vi "MenuBar Visable.vi"(8 "error in (no error)":errorcluster, 10 "Disabled":T1(ring)=enum."Disabled and Grayed Out", 11 "Main in":refnum<class "Main.lvclass">) -> (0 "error out":errorcluster, 3 "Main out":refnum<class "Main.lvclass">)   [LabVIEW 2023, in "GUI.lvlib" / "Main.lvlib" / "Main.lvclass"]
uses:
  Main.lvclass
  Main.lvclass/Main.ctl
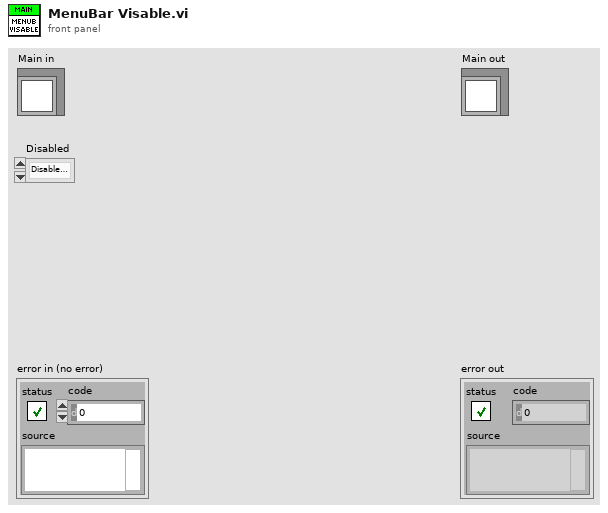
[diagram p1: front panel]
types:
  T1 = enum8{"Enabled", "Disabled", "Disabled and Grayed Out"}
  T2 = typedef "GUI.lvlib/Main.App.Cluster.ctl" = cluster{"Sidebar":refnum<vi>, "Menubar":refnum<vi>, "Log in And Out":refnum<vi>, "User Level":refnum<vi>, "User":refnum<vi>, "Sub Panel":refnum<vi>, "Panel Name":refnum<vi>, "Menu":refnum<vi>, "Close":refnum<vi>}
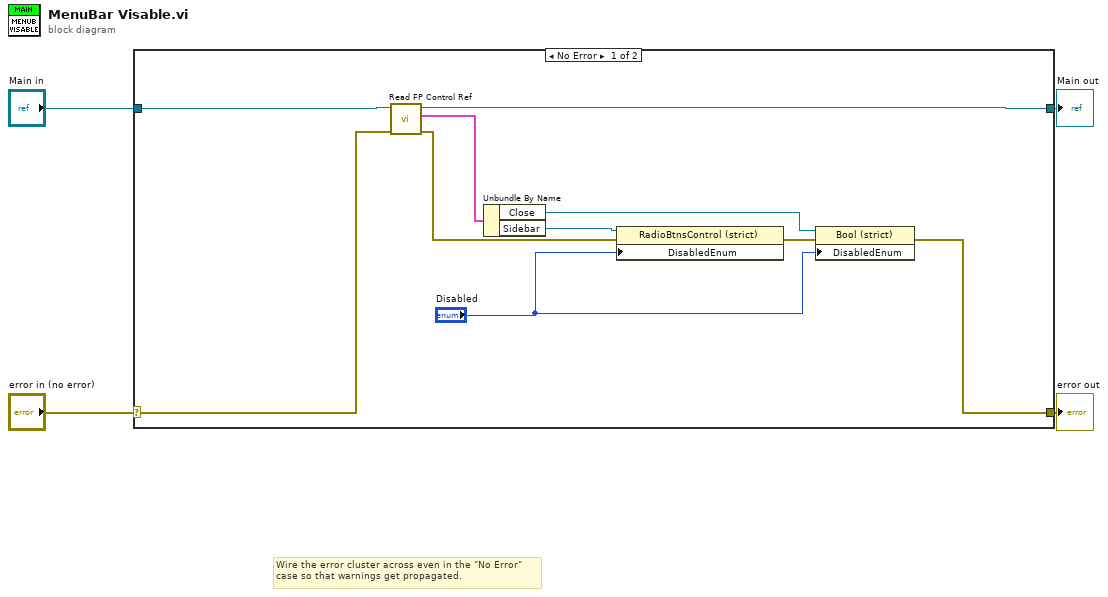
[diagram p0: block diagram]
diagram:
  # "Wire the error cluster across even in the \"No Error\"\ncase so that warnings get propagated."
  n1 = case shown="No Error" "error in (no error)" {
    selector: "error in (no error)" -> [w13 w16]
    tunnel: [w6 w16] -> w3
    tunnel: [w12 w15] -> w1
    tunnel: "Main in" -> [w14 w15]
    frame No Error {
      n2 = call "Read FP Control Ref.vi"("error in (no error)"=w13, "Main in"=w14) -> ("error out"=w9:errorcluster, "FP Control Ref"=w11:T2, "Main out"=w12:refnum<class "Main.lvclass">)  [unwired: 7 in]
      n3 = Unbundle By Name(w11) -> ("Close"=w8:refnum<vi>, "Sidebar"=w10:refnum<vi>)
      n4 = property class="RadioBtnsControl (strict)"(reference=w10, error in=w9, "DisabledEnum"="Disabled") -> (error out=w7:errorcluster)  [unwired: 1 out]
      n5 = property class="Bool (strict)"(reference=w8, error in=w7, "DisabledEnum"="Disabled") -> (error out=w6:errorcluster)  [unwired: 1 out]
    }
    frame Error {
    }
  }
  "error out" <- w3
  "Main out" <- w1
